vi "Replace Cell.vi"(8 "error in (no error)":errorcluster, 9 "Index":i32, 10 "Schedule Cell":refnum<class "Schedule Cell.lvclass">, 11 "Schedule in":refnum<class "Schedule.lvclass">) -> (0 "error out":errorcluster, 3 "Schedule out":refnum<class "Schedule.lvclass">)   [LabVIEW 2020, in "CIRCUS_uServices.lvlib" / "Run Utilities.lvlib" / "Schedule.lvclass"]
uses:
  Schedule.lvclass
  Schedule.lvclass/Schedule.ctl
  Cell/Schedule Cell.lvclass
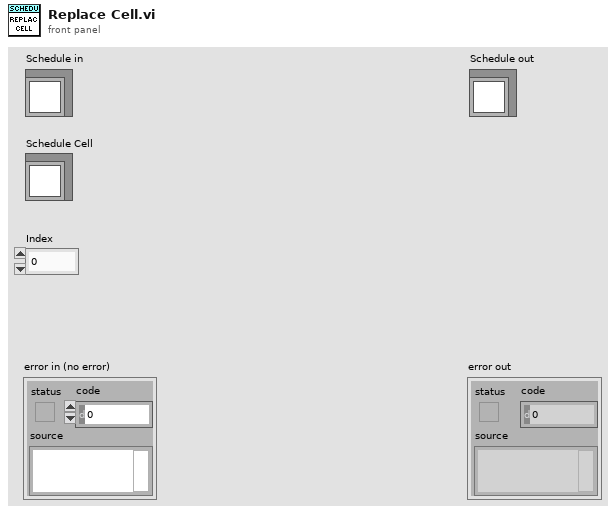
[diagram p1: front panel]
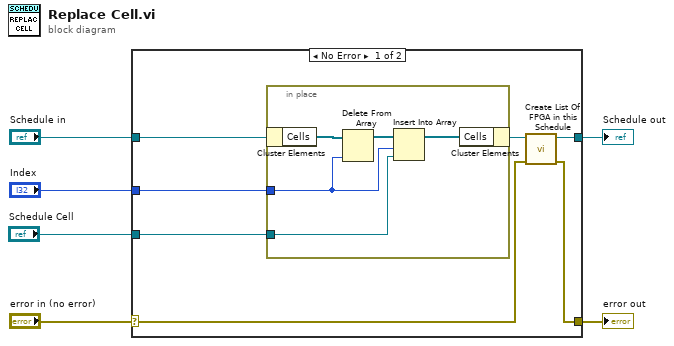
[diagram p0: block diagram]
diagram:
  n1 = case shown="No Error" "error in (no error)" {
    selector: "error in (no error)" -> [w8 w20]
    tunnel: [w7 w20] -> w5
    tunnel: [w9 w19] -> w3
    tunnel: "Schedule in" -> [w13 w19]
    tunnel: "Schedule Cell" -> [w12 _]
    tunnel: "Index" -> [w11 _]
    frame No Error {
      n2 = in-place {
        in-place-border: w12 -> [w14]
        in-place-border: w11 -> [w15]
        n3 = in-place-cluster #1(w13) -> ("Cells"=w18:refnum<class "Schedule Cell.lvclass">[])
        n4 = Delete From Array(array=w18, index=w15) -> (array with subset deleted=w17:refnum<class "Schedule Cell.lvclass">[])  [unwired: 1 in, 1 out]
        n5 = Insert Into Array(array=w17, index=w15, new element=w14) -> (w16:refnum<class "Schedule Cell.lvclass">[])
        n6 = in-place-cluster #1("Cells"=w16) -> (w10:refnum<class "Schedule.lvclass">)
      }
      n7 = call-dynamic "Create List Of FPGA in this Schedule.vi"("error in (no error)"=w8, "Schedule in"=w10) -> ("error out"=w7:errorcluster, "Schedule out"=w9:refnum<class "Schedule.lvclass">)  [unwired: 8 in]
    }
    frame Error {
    }
  }
  "error out" <- w5
  "Schedule out" <- w3
